vi "Tracer Gas Lite.vi"() -> ()   [LabVIEW 2016]
uses:
  <vilib>/Instr/_visa.llb/VISA Flush IO Buffer Mask.ctl
  <vilib>/Analysis/baseanly.llb/Mean (DBL).vi
  <vilib>/Analysis/NI_AALBase.lvlib
panel:
  in  "Reset AVG":bool
  out "Airflow":waveform(dbl)(graph)
  out "Airflow (SCFM)":dbl
  out "Base GA data":T1
  in  "Tab Control":T2(tab)
  out "CO2 Baseline (PPM)":dbl
  out "B-COMMS?":bool
  in  "Baseline Gas Analyzer COM PORT":refnum<visa-resource-name>
  out "set point (slpm)":dbl
  out "mass flow (slpm)":dbl
  out "CO2 (PPM)":dbl
  out "Inj-comms?":bool
  out "P-COMMS?":bool
  in  "Start new filename":bool
  out "Current time":timestamp format="%<%H:%M:%S>T"
  in  "Shut off injection":bool
  in  "Set point (slpm)":dbl
  in  "Pulse Gas Analyzer COM PORT":refnum<visa-resource-name>
  out "Gas analyzer chart":waveform(dbl)[](graph)
  in  "Reset valves":bool
  in  "Valve 3":bool
  in  "Valve 2":bool
  in  "Valve 1":bool
  in  "Zero now":bool
  in  "Bypass warmup":bool
  out "Zeroing":bool
  out "Warming up":bool
  out "Zero timer":dbl format="%<%H:%M:%S>t"
  out "Warm up timer":dbl format="%<%H:%M:%S>t"
  in  "Injector COM PORT":refnum<visa-resource-name>
  out "path":path
  out "file name":string
  in  "Get Ing AVG":bool
  out "Ing AVG Size":i32
  in  "Get CO2 AVG":bool
  out "CO2 AVG Size":i32
  out "Active Valve":string
  out "Injector chart":waveform(dbl)[](graph)
  in  "Estimated Usable Weight (lbs)":dbl
  out "Estimated test time avialable (hh:mm:ss)":dbl=nan format="%<%H:%M:%S>t"
  in  "Injection rate (slpm)":dbl
  in  "Actual Baseline CO2 Concentration (ppm)":dbl
  in  "Actual Measured CO2 Concentration (ppm)":dbl
  in  "Actual Injection Rate (slpm)":dbl
  out "Calculated Flow (scfm)":dbl
  out "Uncertainty (+/- scfm)":dbl=nan
  out "Uncertainty (%)":dbl=nan
  in  "Ambient CO2 (ppm)":dbl=450.0
  in  "Target CO2 Concentration (ppm)":dbl=1500.0
  in  "Estimated Flow (scfm)":dbl=5000.0
  out "Estimated Injection Rate (slpm)":dbl=148.66204162537164
  in  "Temperature override":bool
  out "Injector status":cluster{"[1]":dbl, "[2]":dbl}(graph)
  out "Gas analyzer status":T3(graph)
  out "Boolean":bool
  out "Inj. options":u16(ring) items=["Default", "Pass Set Point", "Reset"]
  out "Injector warm up":T3(graph)
  out "Gas analyzer warm up":dbl[][](graph)
  in  "Override":bool
  in  "Enum":T4(ring)
  out "Current value":T4(ring)
  out "GA data":T1
  out "injector data":T5
  out "error codes":string
  out "Result path":path
  out "write GA data?":bool
  out "write inj data?":bool
  in  "Temp In Range?":bool
  in  "upper limit":dbl=40.0
  in  "lower limit":dbl=5.0
  # "Calculate injection rate based on baseline CO2, target CO2, and estimated airflow rate."
  # "Time available for testing based on the mass of CO2 inside the tank and the desired injection rate."
  # "Calculate airflow rate and uncertainty based on actual injection rate, baseline CO2, and measured CO2."
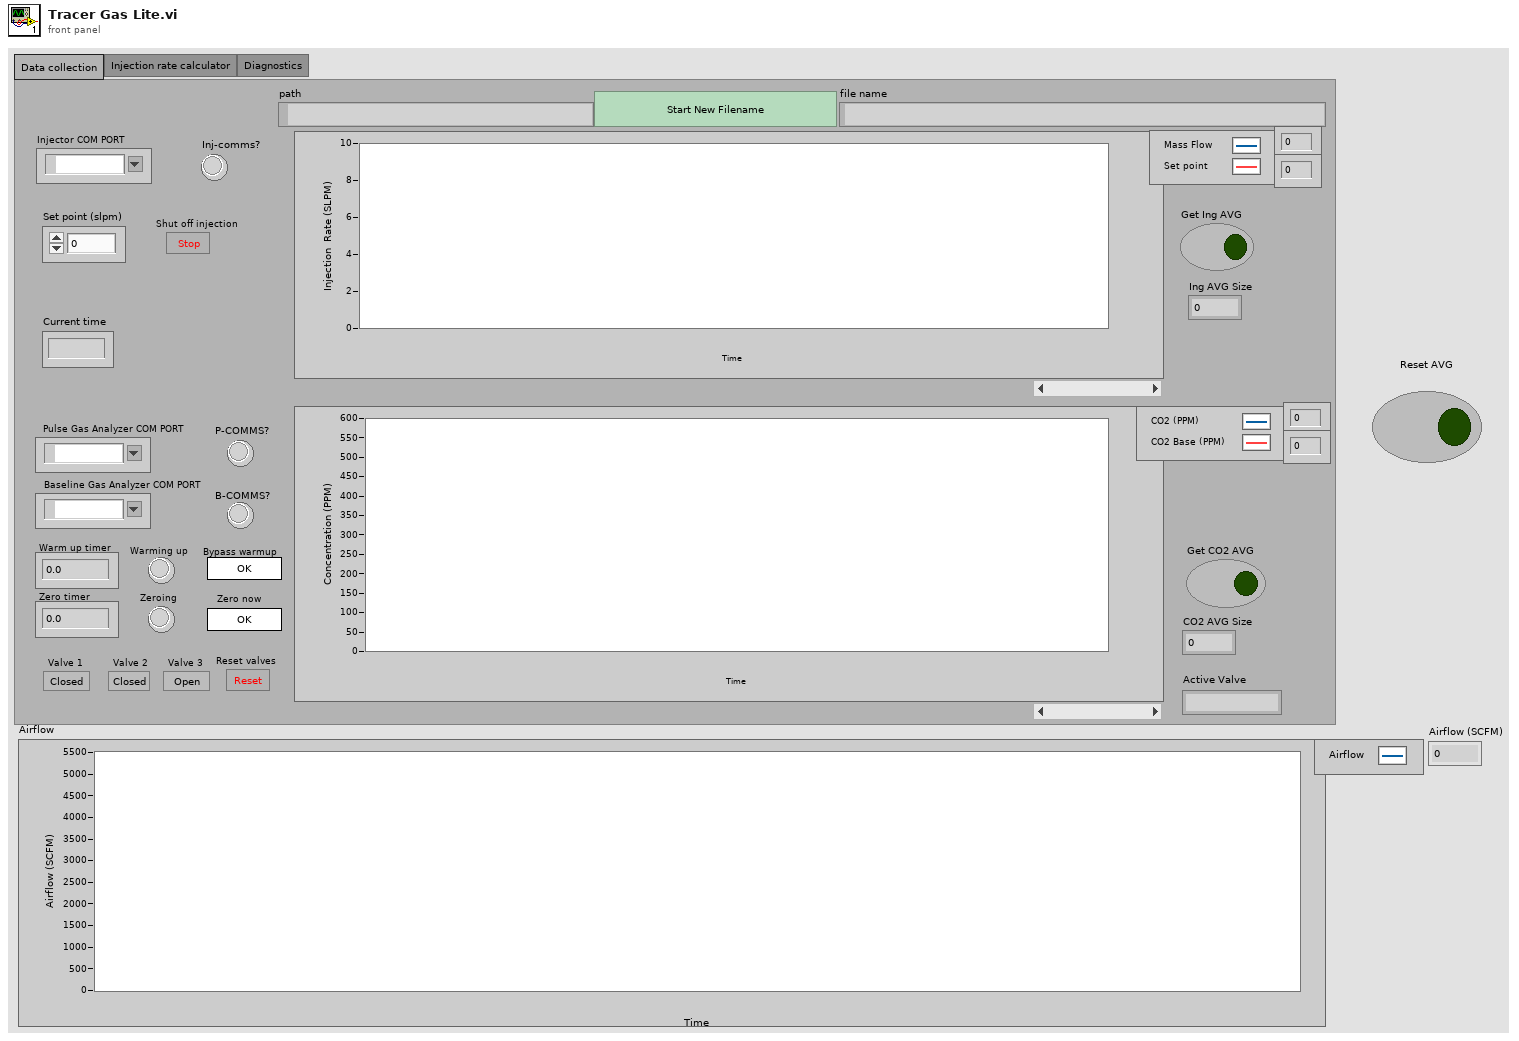
[diagram p1: front panel]
types:
  T1 = cluster{"seconds since 1Jan1904":timestamp, "date string":string, "time string":string, "Array[3]":string, "Array[4]":string, "Array[7]":string, "Array[8]":string, "Array[9]":string}
  T2 = enum32{"Data collection", "Injection rate calculator", "Diagnostics"}
  T3 = cluster{"[0]":dbl, "[1]":dbl, "[2]":dbl, "[3]":dbl, "[4]":dbl, "[5]":dbl, "[6]":dbl, "[7]":dbl, "[8]":dbl}
  T4 = enum16{"Startup", "Warm up", "Poll/Zero", "Run", "Shutdown"}
  T5 = cluster{"seconds since 1Jan1904":timestamp, "date string":string, "time string":string, "[1]":dbl, "[2]":dbl, "[3]":dbl, "[4]":dbl, "[5]":dbl}
  T6 = enum16{"Time", "Zero", "Poll", "Read Buffer", "Set Stream", "Set Poll", "Pump On", "Pump Off", "Set Zero Timing", "Set CO2 Avg.", "Set Measument Format", "Startup Zero Off", "Statup Zero On", "Short Zero Duration", "Set Scaling Factor", "Set Dec Points", "Set Low CO2 Alarm", "Set Analog Output Type", "Set Analog Output Scaling", "Set Data Valid Pin I/O", "Save Current Settings", "Restore Default Settings", "Display Current Settings", "Medium Zero Duration", "Long Zero Duration"}
  T7 = enum16{"Poll", "Set Stream", "Set Poll", "Define Set Point", "Gas Select", "Set P Gain", "Set D Gain", "Get P Gain", "Get D Gain", "Assign New Addess", ""}
  T8 = typedef "VISA Flush IO Buffer Mask.ctl" = u16
  T9 = cluster{"[0]":string, "[1]":string, "[2]":string, "[3]":string, "[4]":string}
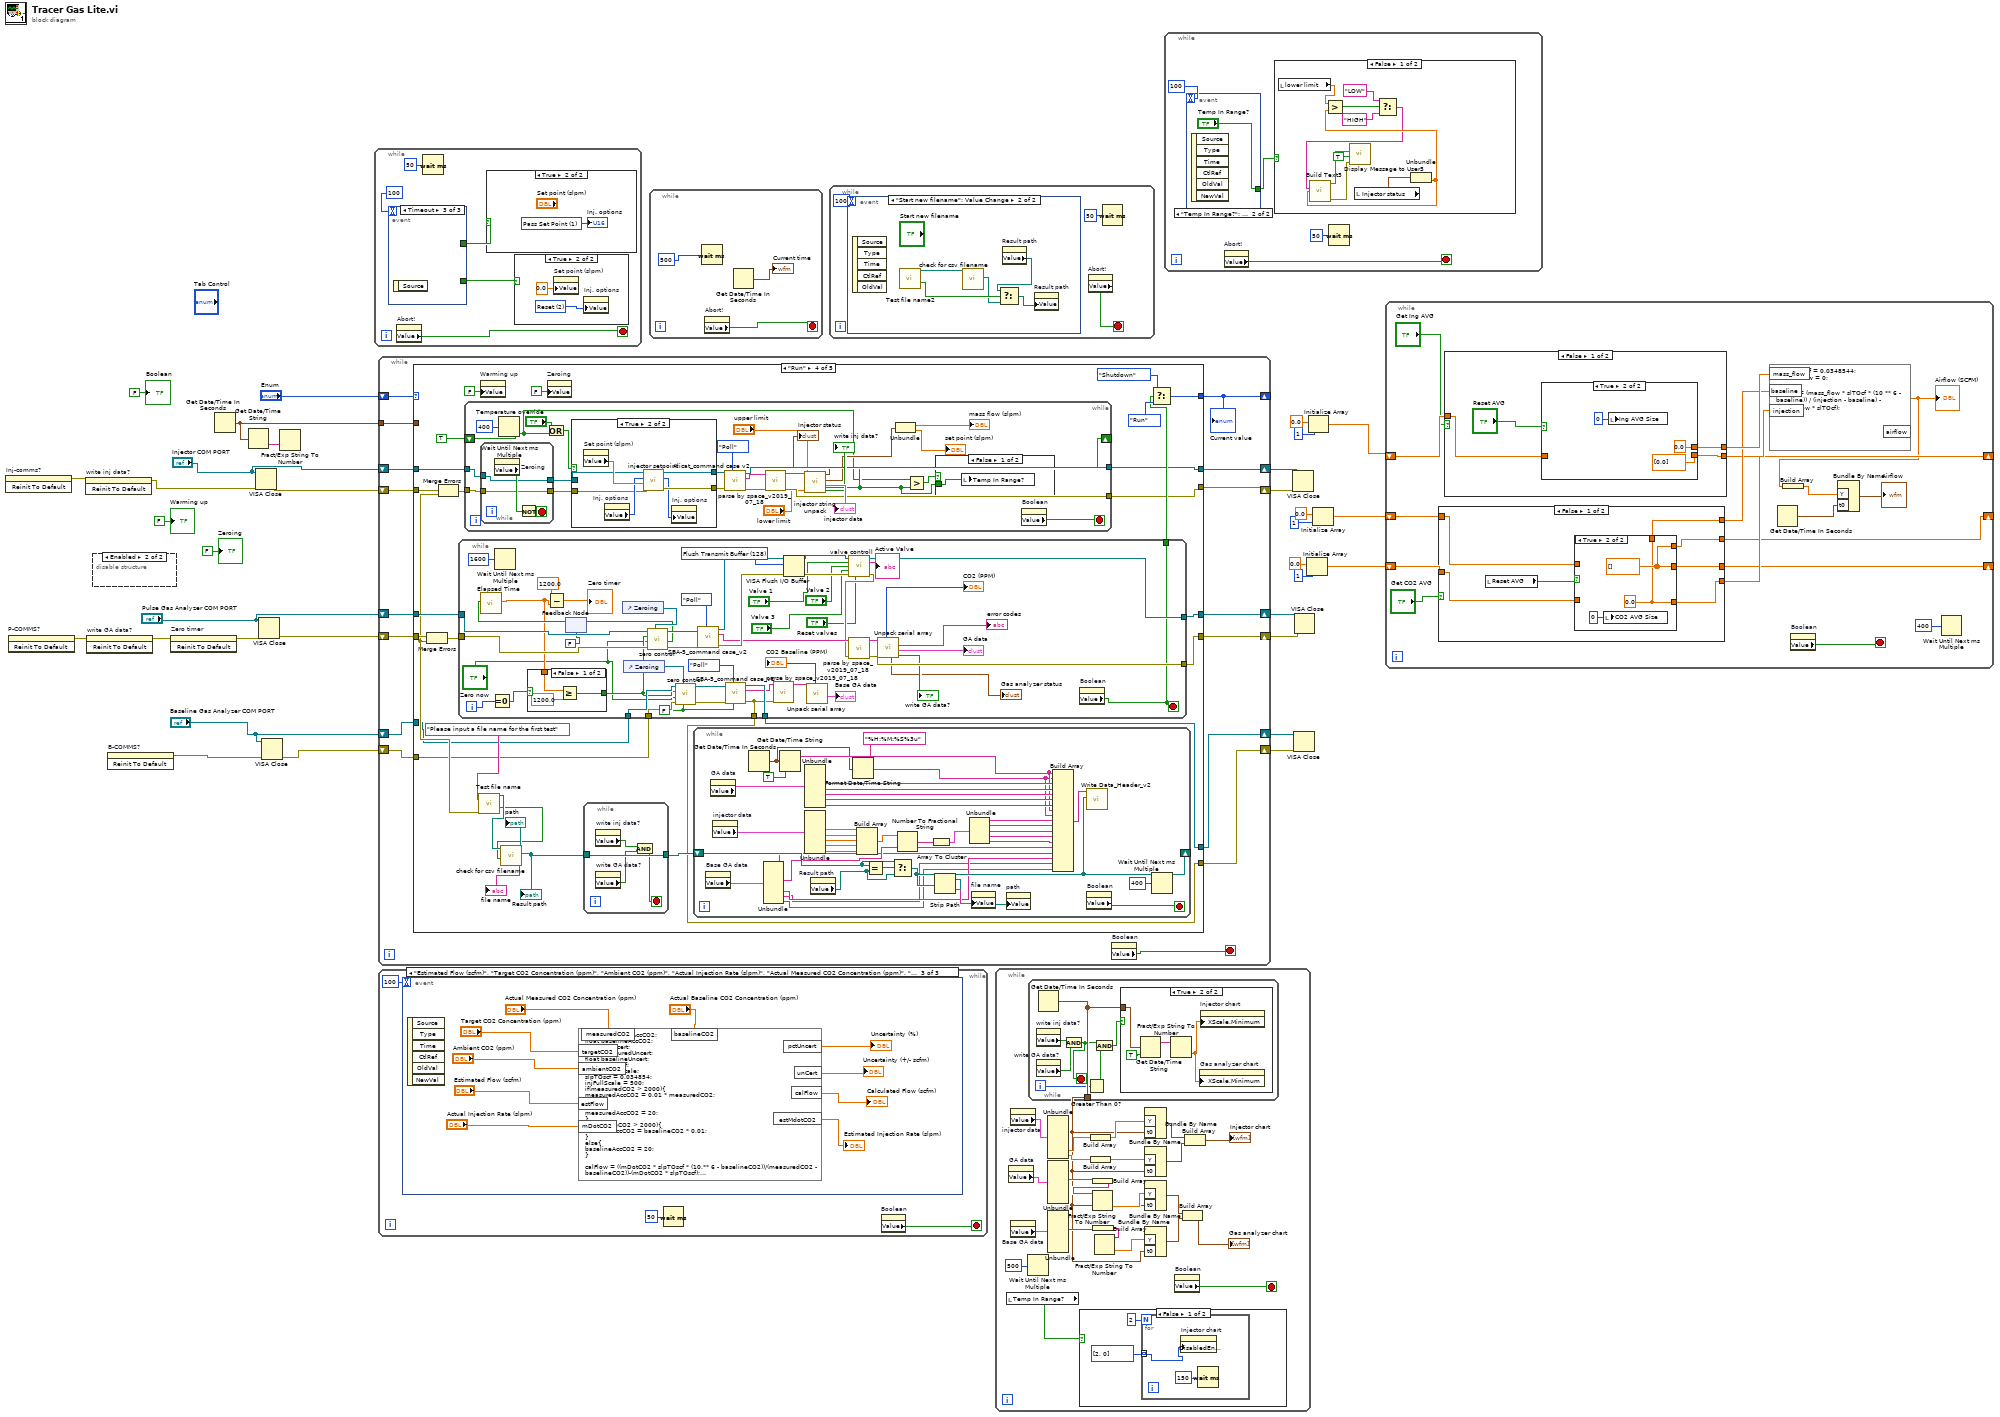
[diagram p0: block diagram]
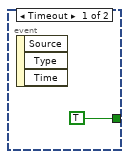
[diagram p3: hidden frame]
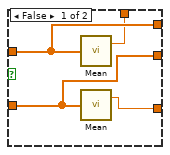
[diagram p4: hidden frame]
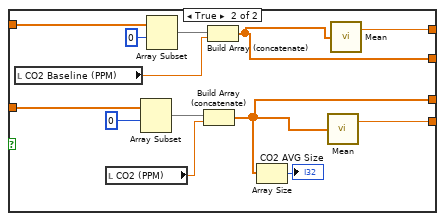
[diagram p5: hidden frame]
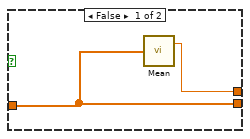
[diagram p6: hidden frame]
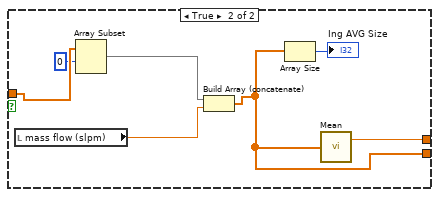
[diagram p7: hidden frame]
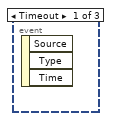
[diagram p10: hidden frame]
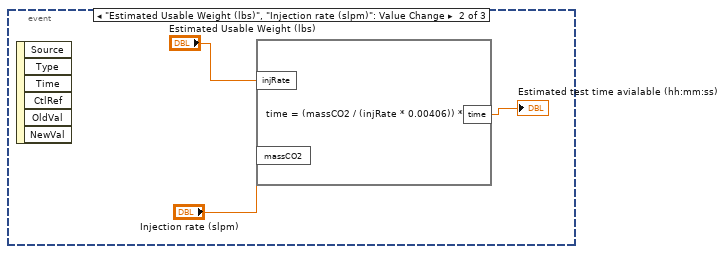
[diagram p11: hidden frame]
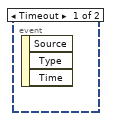
[diagram p12: hidden frame]
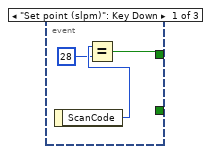
[diagram p15: hidden frame]
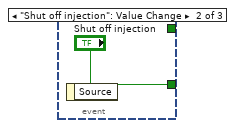
[diagram p16: hidden frame]
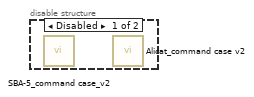
[diagram p17: hidden frame]
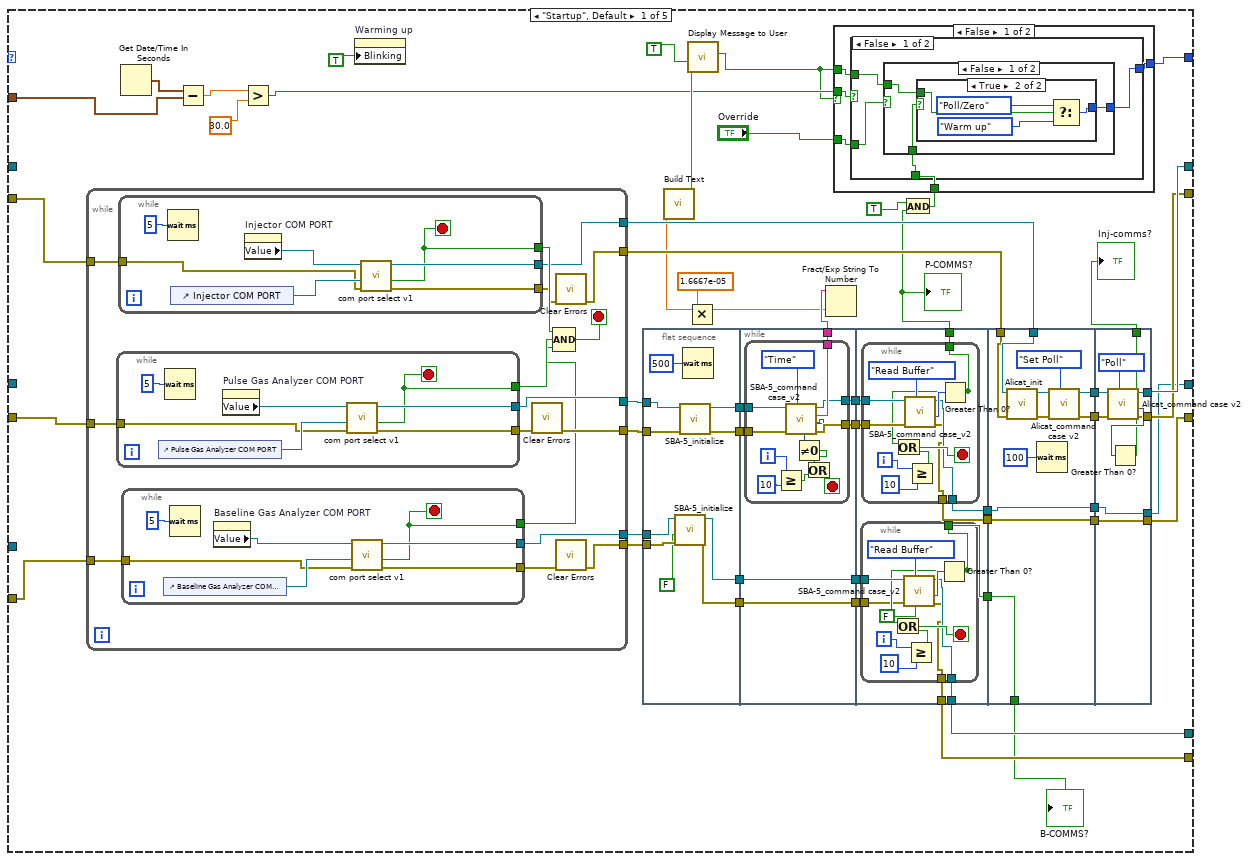
[diagram p18: hidden frame]
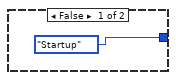
[diagram p19: hidden frame]
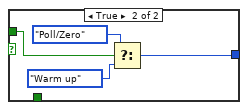
[diagram p20: hidden frame]
diagram:
  n1 = invoke on="Inj-comms?" class="Bool (strict)" method="Reinit To Default"() -> (error out=w16:errorcluster)  [unwired: 3 in, 2 out]
  n2 = invoke on="P-COMMS?" class="Bool (strict)" method="Reinit To Default"() -> (error out=w19:errorcluster)  [unwired: 3 in, 2 out]
  n3 = invoke on="write inj data?" class="Bool (strict)" method="Reinit To Default"(error in=w16) -> (error out=w15:errorcluster)  [unwired: 2 in, 2 out]
  n4 = invoke on="write GA data?" class="Bool (strict)" method="Reinit To Default"(error in=w19) -> (error out=w18:errorcluster)  [unwired: 2 in, 2 out]
  n5 = disable-structure shown="Enabled" {
    frame Disabled {
      n6 = call "SBA-5_command case_v2.vi"() -> ()  [unwired: 8 in, 4 out]
      n7 = call "Alicat_command case v2.vi"() -> ()  [unwired: 8 in, 4 out]
    }
    frame Enabled {
    }
  }
  n8 = invoke on="B-COMMS?" class="Bool (strict)" method="Reinit To Default"() -> (error out=w11:errorcluster)  [unwired: 3 in, 2 out]
  n9 = invoke on="Zero timer" class="DigNum (strict)" method="Reinit To Default"(error in=w18) -> (error out=w17:errorcluster)  [unwired: 2 in, 2 out]
  n10 = Get Date/Time In Seconds() -> (seconds since 1Jan1904=w28:timestamp)
  n11 = Get Date/Time String(seconds (now)=w28) -> (time string=w27:string)  [unwired: 2 in, 1 out]
  n12 = VISA Close(VISA resource name="Injector COM PORT", error in (no error)=w15) -> (error out=w29:errorcluster)
  n13 = VISA Close(VISA resource name="Pulse Gas Analyzer COM PORT", error in (no error)=w17) -> (error out=w32:errorcluster)
  n14 = VISA Close(VISA resource name="Baseline Gas Analyzer COM PORT", error in (no error)=w11) -> (error out=w14:errorcluster)
  n15 = Fract/Exp String To Number(string=w27) -> ()  [unwired: 3 in, 2 out]
  n16 = while {
    stop <- w35 stop-if-true
    n17 = event shown="[2] Timeout" {
      selector: _ -> [_ _ _]
      dyn-events: _ -> [_ _ _]
      timeout: 100 -> [_ _ _]
      tunnel: [_ "Shut off injection" _] -> w37
      tunnel: [w42 _ _] -> w34
      event "Set point (slpm)": Key Down {
        n18 = event-data() -> ("ScanCode"=w44:i16)  [unwired: 1 in]
        n19 = Equal?(x=w44, y=i16 28) -> (x = y?=w42:bool)
      }
      event "Shut off injection": Value Change {
        n20 = event-data() -> ()  [unwired: 1 in, 1 out]
      }
      event Timeout {
        n21 = event-data() -> ()  [unwired: 1 in, 1 out]
      }
    }
    n22 = property on="Abort!" class="Bool (strict)"() -> ("Value"=w35:bool)  [unwired: 2 in, 2 out]
    n23 = Wait (ms)(milliseconds to wait=u32 50) -> ()  [unwired: 1 out]
    n24 = case shown="True" w34 {
      frame False {
      }
      frame True {
        w41 = u16 1 items=["Default", "Pass Set Point", "Reset"] ("Menu Ring")
        "Inj. options" <- w41
      }
    }
    n25 = case shown="True" w37 {
      frame False {
      }
      frame True {
        w40 = u16 2 items=["Default", "Pass Set Point", "Reset"] ("Menu Ring")
        n26 = property on="Set point (slpm)" class="DigNum (strict)"("Value"=0.0 ("Set point (slpm)")) -> ()  [unwired: 2 in, 2 out]
        n27 = property on="Inj. options" class="Ring (strict)"("Value"=w40) -> ()  [unwired: 2 in, 2 out]
      }
    }
  }
  n28 = while {
    shift-right: [w57] -> w24
    shift-left: "Pulse Gas Analyzer COM PORT" -> [w60]
    shift-right: [w56] -> w23
    shift-left: w32 -> [w59]
    shift-right: [w58] -> w26
    shift-left: "Injector COM PORT" -> [w55]
    shift-right: [w51] -> _
    shift-left: "Enum" -> [w61]
    shift-right: [w53] -> w25
    shift-left: w29 -> [w54]
    tunnel: w28 -> [w52]
    shift-right: [w47] -> w13
    shift-left: "Baseline Gas Analyzer COM PORT" -> [w49]
    shift-right: [w46] -> w12
    shift-left: w14 -> [w48]
    stop <- w50 stop-if-true
    n29 = case shown="\"Run\"" w61 {
      tunnel: w60 -> [_ w283 w337 w406 w558]
      tunnel: w59 -> [w111 w286 w340 w394 w557]
      tunnel: [w95 w276 w346 w384 w556] -> w58
      tunnel: [w94 w277 w345 w385 w555] -> w53
      tunnel: [w69 w274 w338 w404 w558] -> w57
      tunnel: [w66 w275 w334 w405 w557] -> w56
      tunnel: w55 -> [_ w281 w346 w397 w556]
      tunnel: w54 -> [w101 w282 w345 w396 w555]
      tunnel: w52 -> [w92 _ _ _ _]
      tunnel: [w88 T4."Poll/Zero" ("Enum") T4."Run" ("Enum") w400 T4."Shutdown" ("Enum")] -> w51
      tunnel: w49 -> [_ w272 w332 w382 w554]
      tunnel: w48 -> [w78 w271 w331 w381 w553]
      tunnel: [w65 w269 w330 w380 w554] -> w47
      tunnel: [w64 w270 w329 w379 w553] -> w46
      frame "Startup", Default {
        n30 = while {
          tunnel: [w240] -> w104
          tunnel: w111 -> [w245]
          tunnel: [w241] -> w105
          tunnel: [w239] -> w110
          tunnel: [w238] -> w109
          tunnel: w101 -> [w237]
          tunnel: w78 -> [w236]
          tunnel: [w233] -> w77
          tunnel: [w232] -> w76
          stop <- w247 stop-if-true
          n31 = while {
            tunnel: [w268] -> w246
            tunnel: w245 -> [w264]
            tunnel: [w263] -> w238
            tunnel: [w262] -> w242
            stop <- w262 stop-if-true
            n32 = control-ref of="Pulse Gas Analyzer COM PORT"() -> (w266:refnum<vi>)
            n33 = Wait (ms)(milliseconds to wait=u32 5) -> ()  [unwired: 1 out]
            n34 = property on="Pulse Gas Analyzer COM PORT" class="VISAName"() -> ("Value"=w265:refnum<visa-resource-name>)  [unwired: 2 in, 2 out]
            n35 = call "com port select v1.vi"("error in (no error)"=w264, "Ctl Refnum"=w266, "VISA resource name in"=w265) -> ("error out"=w268:errorcluster, "COM PORT?"=w262:bool, "VISA resource name out"=w263:refnum<visa-resource-name>)  [unwired: 6 in]
          }
          n36 = while {
            tunnel: [w258] -> w243
            tunnel: [w257] -> w241
            tunnel: [w256] -> w244
            tunnel: w237 -> [w255]
            stop <- w256 stop-if-true
            n37 = Wait (ms)(milliseconds to wait=u32 5) -> ()  [unwired: 1 out]
            n38 = control-ref of="Injector COM PORT"() -> (w261:refnum<vi>)
            n39 = property on="Injector COM PORT" class="VISAName"() -> ("Value"=w259:refnum<visa-resource-name>)  [unwired: 2 in, 2 out]
            n40 = call "com port select v1.vi"("error in (no error)"=w255, "Ctl Refnum"=w261, "VISA resource name in"=w259) -> ("error out"=w258:errorcluster, "COM PORT?"=w256:bool, "VISA resource name out"=w257:refnum<visa-resource-name>)  [unwired: 6 in]
          }
          n41 = while {
            tunnel: [w254] -> w235
            tunnel: w236 -> [w251]
            tunnel: [w250] -> w233
            tunnel: [w249] -> w234
            stop <- w249 stop-if-true
            n42 = control-ref of="Baseline Gas Analyzer COM PORT"() -> (w252:refnum<vi>)
            n43 = Wait (ms)(milliseconds to wait=u32 5) -> ()  [unwired: 1 out]
            n44 = property on="Baseline Gas Analyzer COM PORT" class="VISAName"() -> ("Value"=w248:refnum<visa-resource-name>)  [unwired: 2 in, 2 out]
            n45 = call "com port select v1.vi"("error in (no error)"=w251, "Ctl Refnum"=w252, "VISA resource name in"=w248) -> ("error out"=w254:errorcluster, "COM PORT?"=w249:bool, "VISA resource name out"=w250:refnum<visa-resource-name>)  [unwired: 6 in]
          }
          n46 = call <vilib>:"Clear Errors.vi"("error in (no error)"=w246) -> ("error out"=w239:errorcluster)  [unwired: 5 in, 1 out]
          n47 = Compound Arithmetic op=AND(w244, w242, w234) -> (w247:bool)
          n48 = call <vilib>:"Clear Errors.vi"("error in (no error)"=w243) -> ("error out"=w240:errorcluster)  [unwired: 5 in, 1 out]
          n49 = call <vilib>:"Clear Errors.vi"("error in (no error)"=w235) -> ("error out"=w232:errorcluster)  [unwired: 5 in, 1 out]
        }
        n50 = Get Date/Time In Seconds() -> (seconds since 1Jan1904=w93:timestamp)
        n51 = Subtract(x=w93, y=w92) -> (x-y=w91:dbl)
        n52 = Greater?(x=w91, y=30.0) -> (0:w89:bool)
        n53 = property on="Warming up" class="Bool (strict)"("Blinking"=TRUE) -> ()  [unwired: 2 in, 2 out]
        n54 = flat-sequence {
          tunnel: w110 -> [w159]
          tunnel: w109 -> [w158]
          tunnel: [w156] -> w108
          tunnel: [w155] -> w107
          tunnel: w77 -> [w154]
          tunnel: w76 -> [w153]
          tunnel: [w152] -> w74
          tunnel: [w151] -> w72
          tunnel: w108 -> [w166]
          tunnel: w107 -> [w165]
          tunnel: [w164] -> w103
          tunnel: [w163] -> w100
          tunnel: [w162] -> w99
          tunnel: [w161] -> w75
          tunnel: w74 -> [w161]
          tunnel: [w160] -> w73
          tunnel: w72 -> [w160]
          tunnel: w100 -> [w188]
          tunnel: w99 -> [w187]
          tunnel: [w186] -> w79
          tunnel: w75 -> [w185]
          tunnel: w73 -> [w184]
          tunnel: [w183] -> w70
          tunnel: [w182] -> w67
          tunnel: [w181] -> w65
          tunnel: [w180] -> w64
          tunnel: [w179] -> w62
          tunnel: w105 -> [w222]
          tunnel: w104 -> [w221]
          tunnel: [w219] -> w97
          tunnel: [w220] -> w96
          tunnel: [w214] -> w71
          tunnel: w70 -> [w214]
          tunnel: [w213] -> w68
          tunnel: w67 -> [w213]
          tunnel: [w212] -> w63
          tunnel: w62 -> [w212]
          tunnel: w97 -> [w230]
          tunnel: w96 -> [w231]
          tunnel: [w227] -> w80
          tunnel: [w226] -> w95
          tunnel: [w225] -> w94
          tunnel: w71 -> [w224]
          tunnel: [w224] -> w69
          tunnel: w68 -> [w223]
          tunnel: [w223] -> w66
          frame #0 {
            n55 = call "SBA-5_initialize.vi"("error in (no error)"=w153, "Valve control"=FALSE, "VISA resource name"=w154) -> ("error out"=w151:errorcluster, "VISA resource name out"=w152:refnum<visa-resource-name>)  [unwired: 7 in]
            n56 = call "SBA-5_initialize.vi"("error in (no error)"=w159, "VISA resource name"=w158) -> ("error out"=w155:errorcluster, "VISA resource name out"=w156:refnum<visa-resource-name>)  [unwired: 8 in]
            n57 = Wait (ms)(milliseconds to wait=u32 500) -> ()  [unwired: 1 out]
          }
          frame #1 {
            n58 = while {
              tunnel: w166 -> [w177]
              tunnel: w165 -> [w176]
              tunnel: [w175] -> w164
              tunnel: [w174] -> w163
              tunnel: [w173] -> w162
              i -> [w172]
              stop <- w167 stop-if-true
              n59 = Greater Or Equal?(x=w172, y=10) -> (x >= y?=w170:bool)
              n60 = call "SBA-5_command case_v2.vi"("Case"=T6."Time", "error in (no error)"=w176, "VISA resource name"=w177) -> ("error out"=w173:errorcluster, "bytes out"=w168:u32, "StringFromSBA-5"=w175:string, "dup VISA resource name"=w174:refnum<visa-resource-name>)  [unwired: 5 in]
              n61 = Not Equal To 0?(x=w168) -> (x != 0?=w169:bool)
              n62 = Or(x=w169, y=w170) -> (x .or. y?=w167:bool)
            }
          }
          frame #2 {
            n63 = while {
              tunnel: w185 -> [w199]
              tunnel: [w193] -> w179
              tunnel: [w192] -> w181
              tunnel: [w191] -> w180
              tunnel: w184 -> [w190]
              i -> [w196]
              stop <- w197 stop-if-true
              n64 = call "SBA-5_command case_v2.vi"("Valve control"=FALSE, "Case"=T6."Read Buffer", "error in (no error)"=w190, "VISA resource name"=w199) -> ("error out"=w191:errorcluster, "bytes out"=w198:u32, "dup VISA resource name"=w192:refnum<visa-resource-name>)  [unwired: 4 in, 1 out]
              n65 = Greater Or Equal?(x=w196, y=10) -> (x >= y?=w194:bool)
              n66 = Greater Than 0?(x=w198) -> (x > 0?=w193:bool)
              n67 = Or(x=w193, y=w194) -> (x .or. y?=w197:bool)
            }
            n68 = while {
              tunnel: w188 -> [w210]
              tunnel: w187 -> [w209]
              tunnel: [w203] -> w186
              tunnel: [w202] -> w183
              tunnel: [w201] -> w182
              i -> [w206]
              stop <- w207 stop-if-true
              n69 = call "SBA-5_command case_v2.vi"("Case"=T6."Read Buffer", "error in (no error)"=w209, "VISA resource name"=w210) -> ("error out"=w201:errorcluster, "bytes out"=w208:u32, "dup VISA resource name"=w202:refnum<visa-resource-name>)  [unwired: 5 in, 1 out]
              n70 = Greater Or Equal?(x=w206, y=10) -> (x >= y?=w204:bool)
              n71 = Greater Than 0?(x=w208) -> (x > 0?=w203:bool)
              n72 = Or(x=w203, y=w204) -> (x .or. y?=w207:bool)
            }
          }
          frame #3 {
            n73 = call "Alicat_init.vi"("error in (no error)"=w221, "VISA resource name"=w222) -> ("error out"=w217:errorcluster, "VISA resource name out"=w218:refnum<visa-resource-name>)  [unwired: 8 in]
            n74 = Wait (ms)(milliseconds to wait=u32 100) -> ()  [unwired: 1 out]
            n75 = call "Alicat_command case v2.vi"("Case"=T7."Set Poll", "error in (no error)"=w217, "VISA resource name"=w218) -> ("error out"=w220:errorcluster, "dup VISA resource name"=w219:refnum<visa-resource-name>)  [unwired: 5 in, 2 out]
          }
          frame #4 {
            n76 = call "Alicat_command case v2.vi"("Case"=T7."Poll", "error in (no error)"=w231, "VISA resource name"=w230) -> ("error out"=w225:errorcluster, "bytes at port"=w228:u32, "dup VISA resource name"=w226:refnum<visa-resource-name>)  [unwired: 5 in, 1 out]
            n77 = Greater Than 0?(x=w228) -> (x > 0?=w227:bool)
          }
        }
        n78 = Fract/Exp String To Number(string=w103) -> (number=w102:dbl)  [unwired: 3 in, 1 out]
        n79 = Multiply(x=w102, y=1.6667e-05) -> (x*y=w84:dbl)
        n80 = call "Build Text"("minutes"=w84) -> ("Result"=w98:string)  [unwired: 13 in, 1 out]
        n81 = call "Display Message to User"("Enable"=TRUE, "Message"=w98) -> ("Yes"=w81:bool)  [unwired: 8 in, 1 out]
        n82 = And(x=TRUE, y=w79) -> (x .and. y?=w86:bool)
        n83 = case shown="False" w81 {
          tunnel: w89 -> [w116 _]
          tunnel: [w115 T4."Poll/Zero" ("Enum")] -> w88
          tunnel: "Override" -> [w114 _]
          tunnel: w81 -> [w113 _]
          tunnel: w86 -> [w112 _]
          frame False {
            n84 = case shown="False" w116 {
              tunnel: [w118 w134] -> w115
              tunnel: w114 -> [w120 w136]
              tunnel: w113 -> [w119 w135]
              tunnel: w112 -> [w117 w133]
              frame False {
                n85 = case shown="False" w120 {
                  tunnel: w119 -> [w122 w131]
                  tunnel: [w121 w129] -> w118
                  tunnel: w117 -> [w123 _]
                  frame False {
                    n86 = case shown="True" w123 {
                      tunnel: w122 -> [_ w128]
                      tunnel: [T4."Startup" ("Enum") w125] -> w121
                      frame False {
                      }
                      frame True {
                        n87 = Select(t=T4."Poll/Zero" ("Enum"), s=w128, f=T4."Warm up" ("Enum")) -> (s? t:f=w125:T4)
                      }
                    }
                  }
                  frame True {
                    n88 = Select(t=T4."Poll/Zero" ("Enum"), s=w131, f=T4."Warm up" ("Enum")) -> (s? t:f=w129:T4)
                  }
                }
              }
              frame True {
                n89 = case shown="True" w136 {
                  tunnel: w135 -> [w138 w148]
                  tunnel: [w137 w145] -> w134
                  tunnel: w133 -> [w139 _]
                  frame False {
                    n90 = case shown="False" w139 {
                      tunnel: w138 -> [_ w142]
                      tunnel: [T4."Shutdown" ("Enum") w141] -> w137
                      frame False {
                      }
                      frame True {
                        n91 = Select(t=T4."Poll/Zero" ("Enum"), s=w142, f=T4."Warm up" ("Enum")) -> (s? t:f=w141:T4)
                      }
                    }
                  }
                  frame True {
                    n92 = Select(t=T4."Poll/Zero" ("Enum"), s=w148, f=T4."Warm up" ("Enum")) -> (s? t:f=w145:T4)
                  }
                }
              }
            }
          }
          frame True {
          }
        }
        "Inj-comms?" <- w80
        "P-COMMS?" <- w79
        "B-COMMS?" <- w63
      }
      frame "Warm up" {
        n93 = property on="Warm up timer" class="DigNum (strict)"(error in=w286, "Value"=900.0 ("Warm up timer")) -> (error out=w284:errorcluster)  [unwired: 1 in, 1 out]
        n94 = property on="Warming up" class="Bool (strict)"("Blinking"=FALSE) -> (error out=w279:errorcluster)  [unwired: 2 in, 1 out]
        n95 = while {
          tunnel: w284 -> [w317]
          tunnel: w283 -> [w318]
          tunnel: w282 -> [w315]
          tunnel: w281 -> [w314]
          tunnel: [w303] -> w276
          tunnel: [w301] -> w277
          tunnel: [w300] -> w275
          tunnel: [w299] -> w274
          tunnel: w272 -> [w298]
          tunnel: w271 -> [w297]
          tunnel: [w290] -> w269
          tunnel: [w289] -> w270
          stop <- w311 stop-if-true
          n96 = Wait Until Next ms Multiple(millisecond multiple=u32 1600) -> ()  [unwired: 1 out]
          n97 = call "SBA-5_command case_v2.vi"("Case"=T6."Read Buffer", "error in (no error)"=w317, "VISA resource name"=w318) -> ("error out"=w309:errorcluster, "StringFromSBA-5"=w310:string, "dup VISA resource name"=w299:refnum<visa-resource-name>)  [unwired: 5 in, 1 out]
          n98 = call "SBA-5_command case_v2.vi"("Valve control"=FALSE, "Case"=T6."Read Buffer", "error in (no error)"=w297, "VISA resource name"=w298) -> ("error out"=w296:errorcluster, "StringFromSBA-5"=w295:string, "dup VISA resource name"=w290:refnum<visa-resource-name>)  [unwired: 4 in, 1 out]
          n99 = call "Alicat_command case v2.vi"("Case"=T7."Poll", "error in (no error)"=w315, "VISA resource name"=w314) -> ("error out"=w302:errorcluster, "String From Alicat"=w305:string, "dup VISA resource name"=w303:refnum<visa-resource-name>)  [unwired: 5 in, 1 out]
          n100 = call "parse by space_v2019_07_18.vi"("error in (no error)"=w296, "String"=w295) -> ("error out"=w289:errorcluster, "Array"=w294:string[])  [unwired: 8 in]
          n101 = call "parse by space_v2019_07_18.vi"("error in (no error)"=w302, "String"=w305) -> ("error out"=w301:errorcluster, "Array"=w306:string[])  [unwired: 8 in]
          n102 = call "parse by space_v2019_07_18.vi"("error in (no error)"=w309, "String"=w310) -> ("error out"=w300:errorcluster, "Array"=w308:string[])  [unwired: 8 in]
          n103 = Fract/Exp String To Number(string=w306) -> (number=w307:dbl[])  [unwired: 3 in, 1 out]
          n104 = Fract/Exp String To Number(string=w294) -> (number=w292:dbl[])  [unwired: 3 in, 1 out]
          n105 = Fract/Exp String To Number(string=w308) -> (number=w293:dbl[])  [unwired: 3 in, 1 out]
          n106 = Array To Cluster(array=w307) -> (cluster=→"Injector warm up":T3)
          n107 = Build Array(w293, w292) -> (→"Gas analyzer warm up":dbl[][])
          n108 = property on="Warm up timer" class="DigNum (strict)"() -> ("Value"=w312:dbl)  [unwired: 2 in, 2 out]
          n109 = Less Or Equal To 0?(x=w312) -> (x <= 0?=w311:bool)
        }
        n110 = property on="Warming up" class="Bool (strict)"(error in=w279, "Value"=TRUE ("Blinking")) -> ()  [unwired: 1 in, 2 out]
        n111 = while {
          stop <- w323 stop-if-true
          n112 = call "Warm up timing"() -> ("Elapsed Time (s)"=w327:dbl, "Time has Elapsed"=w322:bool)  [unwired: 12 in, 6 out]
          n113 = Wait Until Next ms Multiple(millisecond multiple=u32 500) -> ()  [unwired: 1 out]
          n114 = Compound Arithmetic op=OR(w322, "Bypass warmup") -> (w323:bool)
          n115 = Subtract(x=900.0, y=w327) -> (x-y=w325:dbl)
          n116 = Select(t=0.0, s="Bypass warmup", f=w325) -> (s? t:f=→"Warm up timer":dbl)
        }
      }
      frame "Poll/Zero" {
        n117 = property on="Zeroing" class="Bool (strict)"(error in=w340, "Blinking"=TRUE ("Zeroing")) -> (error out=w336:errorcluster)  [unwired: 1 in, 1 out]
        n118 = property on="Warming up" class="Bool (strict)"("Blinking"=FALSE) -> (error out=w342:errorcluster)  [unwired: 2 in, 1 out]
        n119 = property on="Warming up" class="Bool (strict)"(error in=w342, "Value"=FALSE ("Blinking")) -> ()  [unwired: 1 in, 2 out]
        n120 = while {
          tunnel: w337 -> [w367]
          tunnel: w336 -> [w365]
          tunnel: [w375] -> w338
          tunnel: [w374] -> w335
          i -> [w370]
          stop <- w371 stop-if-true
          n121 = call "SBA-5_command case_v2.vi"("Case"=T6."Set Poll", "error in (no error)"=w365, "VISA resource name"=w367) -> ("error out"=w364:errorcluster, "dup VISA resource name"=w366:refnum<visa-resource-name>)  [unwired: 5 in, 2 out]
          n122 = Wait Until Next ms Multiple(millisecond multiple=u32 1600) -> ()  [unwired: 1 out]
          n123 = call "SBA-5_command case_v2.vi"("Case"=T6."Poll", "error in (no error)"=w364, "VISA resource name"=w366) -> ("error out"=w374:errorcluster, "bytes out"=w376:u32, "dup VISA resource name"=w375:refnum<visa-resource-name>)  [unwired: 5 in, 1 out]
          n124 = Greater?(x=w370, y=5) -> (0:w368:bool)
          n125 = Greater Than 0?(x=w376) -> (x > 0?=w363:bool)
          n126 = property on="P-COMMS?" class="Bool (strict)"("Value"=w363) -> ()  [unwired: 2 in, 2 out]
          n127 = Or(x=w363, y=w368) -> (x .or. y?=w371:bool)
        }
        n128 = while {
          tunnel: w332 -> [w352]
          tunnel: w331 -> [w350]
          tunnel: [w360] -> w330
          tunnel: [w359] -> w329
          i -> [w355]
          stop <- w356 stop-if-true
          w347 = FALSE ("Valve control")
          n129 = call "SBA-5_command case_v2.vi"("Valve control"=w347, "Case"=T6."Set Poll", "error in (no error)"=w350, "VISA resource name"=w352) -> ("error out"=w349:errorcluster, "dup VISA resource name"=w351:refnum<visa-resource-name>)  [unwired: 4 in, 2 out]
          n130 = Wait Until Next ms Multiple(millisecond multiple=u32 1600) -> ()  [unwired: 1 out]
          n131 = call "SBA-5_command case_v2.vi"("Valve control"=w347, "Case"=T6."Poll", "error in (no error)"=w349, "VISA resource name"=w351) -> ("error out"=w359:errorcluster, "bytes out"=w361:u32, "dup VISA resource name"=w360:refnum<visa-resource-name>)  [unwired: 4 in, 1 out]
          n132 = Greater?(x=w355, y=5) -> (0:w353:bool)
          n133 = Greater Than 0?(x=w361) -> (x > 0?=w348:bool)
          n134 = property on="B-COMMS?" class="Bool (strict)"("Value"=w348) -> ()  [unwired: 2 in, 2 out]
          n135 = Or(x=w348, y=w353) -> (x .or. y?=w356:bool)
        }
        n136 = property on="Zeroing" class="Bool (strict)"(error in=w335, "Blinking"=FALSE) -> (error out=w334:errorcluster)  [unwired: 1 in, 1 out]
      }
      frame "Run" {
        n137 = call "Test file name"("prompt"="Please input a file name for the first test") -> ("selected path"=w390:path, "cancelled"=w383:bool, "error out"=w392:errorcluster)  [unwired: 11 in, 1 out]
        n138 = Merge Errors(w394, w392) -> (w393:errorcluster)
        n139 = Merge Errors(w396, w392) -> (w395:errorcluster)
        n140 = while {
          tunnel: w406 -> [w546]
          tunnel: w393 -> [w545]
          tunnel: [w535] -> w405
          tunnel: [w524] -> w404
          tunnel: [w516] -> w401
          tunnel: w382 -> [w513]
          tunnel: w381 -> [w512]
          tunnel: [w503] -> w380
          tunnel: [w502] -> w379
          i -> [w529]
          stop <- w516 stop-if-true
          w500 = FALSE ("Valve control")
          w538 = T8 128 items=["Flush Receive Buffer"=16, "Write Transmit Buffer to Device"=32, "Flush Receive Buffer (No I/O)"=64, "Flush Transmit Buffer"=128] ("Mask")
          n141 = Equal To 0?(x=w529) -> (x = 0?=w528:bool)
          n142 = Wait Until Next ms Multiple(millisecond multiple=u32 1600) -> ()  [unwired: 1 out]
          n143 = feedback #1(FALSE ("Zero reset")) -> (w532:bool)
          n144 = call "Elapsed Time"("Reset"=w532) -> ("Elapsed Time (s)"=w530:dbl)  [unwired: 11 in, 7 out]
          n145 = case shown="False" w528 {
            tunnel: w530 -> [w550 _]
            tunnel: [w549 TRUE] -> w511
            frame False {
              n146 = Greater Or Equal?(x=w550, y=1200.0) -> (x >= y?=w549:bool)
            }
            frame True {
            }
          }
          n147 = Subtract(x=1200.0, y=w530) -> (x-y=→"Zero timer":dbl)
          n148 = control-ref of="Zeroing"() -> (w544:refnum<vi>)
          n149 = control-ref of="Zeroing"() -> (w501:refnum<vi>)
          n150 = call "zero control.vi"("Ctl Refnum"=w544, "error in (no error)"=w545, "Zero now"="Zero now", "Zero timer"=w511, "VISA resource name"=w546) -> ("error out"=w542:errorcluster, "Zero reset"=w533:bool, "VISA resource out"=w543:refnum<visa-resource-name>)  [unwired: 4 in]
          n151 = feedback-in #1(w533) -> ()
          n152 = call "zero control.vi"("Valve control"=w500, "Ctl Refnum"=w501, "error in (no error)"=w512, "Zero now"="Zero now", "Zero timer"=w511, "VISA resource name"=w513) -> ("error out"=w508:errorcluster, "VISA resource out"=w509:refnum<visa-resource-name>)  [unwired: 3 in, 1 out]
          n153 = call "SBA-5_command case_v2.vi"("Case"=T6."Poll", "error in (no error)"=w542, "VISA resource name"=w543) -> ("error out"=w539:errorcluster, "StringFromSBA-5"=w537:string, "dup VISA resource name"=w540:refnum<visa-resource-name>)  [unwired: 5 in, 1 out]
          n154 = call "SBA-5_command case_v2.vi"("Valve control"=w500, "Case"=T6."Poll", "error in (no error)"=w508, "VISA resource name"=w509) -> ("error out"=w502:errorcluster, "StringFromSBA-5"=w499:string, "dup VISA resource name"=w503:refnum<visa-resource-name>)  [unwired: 4 in, 1 out]
          n155 = call "parse by space_v2019_07_18.vi"("error in (no error)"=w502, "String"=w499) -> ("Array"=w506:string[])  [unwired: 8 in, 1 out]
          n156 = VISA Flush I/O Buffer(VISA resource name=w540, mask (16)=w538, error in (no error)=w539) -> (VISA resource name out=w527:refnum<visa-resource-name>, error out=w526:errorcluster)
          n157 = call "Unpack serial array.vi"("Array"=w506) -> ("Cluster 2"=→"Base GA data":T1, "Numeric"=→"CO2 Baseline (PPM)":i32)  [unwired: 4 in, 5 out]
          n158 = call "valve controll.vi"("VISA Refnum in"=w527, "Valve 1"="Valve 1", "Valve 2"="Valve 2", "Valve 3"="Valve 3", "error in (no error)"=w526, "Reset valves"="Reset valves") -> ("VISA Refnum in 2"=w524:refnum<visa-resource-name>, "Active Valve"=→"Active Valve":string, "error out"=w525:errorcluster)  [unwired: 7 in]
          n159 = call "parse by space_v2019_07_18.vi"("error in (no error)"=w525, "String"=w537) -> ("error out"=w535:errorcluster, "Array"=w536:string[])  [unwired: 8 in]
          n160 = call "Unpack serial array.vi"("Array"=w536) -> ("write data?"=→"write GA data?":bool, "Cluster 2"=→"GA data":T1, "Array[10]"=→"error codes":string, "Cluster"=→"Gas analyzer status":T3, "Numeric"=→"CO2 (PPM)":i32)  [unwired: 4 in, 2 out]
          n161 = property on="Boolean" class="Bool (strict)"() -> ("Value"=w516:bool)  [unwired: 2 in, 2 out]
        }
        n162 = while {
          tunnel: w397 -> [w468]
          tunnel: w395 -> [w466]
          tunnel: [w464] -> w385
          tunnel: [w463] -> w384
          shift-right: [w452] -> _
          shift-left: TRUE -> [w451]
          stop <- w462 stop-if-true
          n163 = while {
            tunnel: w468 -> [w495]
            tunnel: [w495] -> w467
            tunnel: w466 -> [w494]
            tunnel: [w494] -> w465
            stop <- w496 stop-if-true
            n164 = property on="Zeroing" class="Bool (strict)"() -> ("Value"=w497:bool)  [unwired: 2 in, 2 out]
            n165 = Not(x=w497) -> (.not. x?=w496:bool)
          }
          n166 = Wait Until Next ms Multiple(millisecond multiple=u32 400) -> ()  [unwired: 1 out]
          n167 = Or(x="Temperature override", y=w451) -> (x .or. y?=w454:bool)
          n168 = case shown="True" w454 {
            tunnel: [w485 w492] -> w476
            tunnel: [w484 w491] -> w475
            tunnel: w467 -> [w482 w488]
            tunnel: w465 -> [w483 w487]
            frame False {
              w480 = u16 2 items=["Default", "Pass Set Point", "Reset"] ("Menu Ring")
              n169 = call "injector setpoint.vi"("error in (no error)"=w483, "Pass setpoint?"=w480, "VISA Refnum in"=w482) -> ("error out"=w484:errorcluster, "MFC options"=w486:u16, "VISA Refnum out"=w485:refnum<visa-resource-name>)  [unwired: 6 in]
              n170 = property on="Set point (slpm)" class="DigNum (strict)"("Value"=0.0 ("Set point (slpm)")) -> ()  [unwired: 2 in, 2 out]
              n171 = property on="Inj. options" class="Ring (strict)"("Value"=w486) -> ()  [unwired: 2 in, 2 out]
            }
            frame True {
              n172 = property on="Set point (slpm)" class="DigNum (strict)"() -> ("Value"=w493:dbl)  [unwired: 2 in, 2 out]
              n173 = property on="Inj. options" class="Ring (strict)"() -> ("Value"=w490:u16)  [unwired: 2 in, 2 out]
              n174 = call "injector setpoint.vi"("error in (no error)"=w487, "set point"=w493, "Pass setpoint?"=w490, "VISA Refnum in"=w488) -> ("error out"=w491:errorcluster, "MFC options"=w489:u16, "VISA Refnum out"=w492:refnum<visa-resource-name>)  [unwired: 5 in]
              n175 = property on="Inj. options" class="Ring (strict)"("Value"=w489) -> ()  [unwired: 2 in, 2 out]
            }
          }
          n176 = call "Alicat_command case v2.vi"("Case"=T7."Poll", "error in (no error)"=w475, "VISA resource name"=w476) -> ("error out"=w473:errorcluster, "String From Alicat"=w472:string, "dup VISA resource name"=w463:refnum<visa-resource-name>)  [unwired: 5 in, 1 out]
          n177 = call "parse by space_v2019_07_18.vi"("error in (no error)"=w473, "String"=w472) -> ("error out"=w464:errorcluster, "Array"=w471:string[])  [unwired: 8 in]
          n178 = call "injector string unpack.vi"("lower limit"="lower limit", "upper limit"="upper limit", "Array"=w471) -> ("write data?"=→"write inj data?":bool, "data out"=→"injector data":T5, "mass flow/setpoint"=w460:cluster{"[4]":dbl, "[5]":dbl}, "pressure/temp"=→"Injector status":cluster{"[1]":dbl, "[2]":dbl}, "Temp In Range?"=w452:bool)  [unwired: 2 in, 2 out]
          n179 = Unbundle(w460) -> ("[4]"=→"mass flow (slpm)":dbl, "[5]"=→"set point (slpm)":dbl)
          n180 = Greater?(x=w451, y=w452) -> (0:w453:bool)
          n181 = case shown="False" w453 {
            tunnel: w452 -> [w478 w479]
            frame False {
              n182 = local write "Temp In Range?"(w478) -> ()
            }
            frame True {
              n183 = property on="Temp In Range?" class="Bool (strict)"("Val(Sgnl)"=w479) -> ()  [unwired: 2 in, 2 out]
            }
          }
          n184 = property on="Boolean" class="Bool (strict)"() -> ("Value"=w462:bool)  [unwired: 2 in, 2 out]
        }
        n185 = property on="Warming up" class="Bool (strict)"("Value"=FALSE ("Warming up")) -> ()  [unwired: 2 in, 2 out]
        n186 = call "check for csv filename.vi"("Canceled?"=w383, "selected path"=w390) -> ("file name"=→"file name":string, "Result path"=w386:path, "stripped path"=→"path":path)  [unwired: 7 in]
        "Result path" <- w386
        n187 = property on="Zeroing" class="Bool (strict)"("Value"=FALSE ("Zeroing")) -> ()  [unwired: 2 in, 2 out]
        n188 = while {
          tunnel: [w410] -> w387
          tunnel: w386 -> [w410]
          stop <- w407 stop-if-true
          n189 = property on="write inj data?" class="Bool (strict)"() -> ("Value"=w408:bool)  [unwired: 2 in, 2 out]
          n190 = property on="write GA data?" class="Bool (strict)"() -> ("Value"=w409:bool)  [unwired: 2 in, 2 out]
          n191 = And(x=w408, y=w409) -> (x .and. y?=w407:bool)
        }
        n192 = while {
          shift-right: [w445] -> _
          shift-left: w387 -> [w449]
          stop <- w420 stop-if-true
          n193 = property on="Base GA data" class="Clust (strict)"() -> ("Value"=w416:T1)  [unwired: 2 in, 2 out]
          n194 = property on="GA data" class="Clust (strict)"() -> ("Value"=w444:T1)  [unwired: 2 in, 2 out]
          n195 = property on="injector data" class="Clust (strict)"() -> ("Value"=w438:T5)  [unwired: 2 in, 2 out]
          n196 = Get Date/Time In Seconds() -> (seconds since 1Jan1904=w419:timestamp)
          n197 = Unbundle(w416) -> ("Array[3]"=w415:string, "Array[4]"=w414:string, "Array[7]"=w413:string, "Array[8]"=w412:string, "Array[9]"=w411:string)  [unwired: 3 out]
          n198 = Get Date/Time String(seconds (now)=w419, want seconds? (F)=TRUE) -> (date string=w422:string)  [unwired: 1 in, 1 out]
          n199 = Unbundle(w444) -> ("Array[3]"=w443:string, "Array[4]"=w442:string, "Array[7]"=w441:string, "Array[8]"=w440:string, "Array[9]"=w439:string)  [unwired: 3 out]
          n200 = Unbundle(w438) -> ("[1]"=w437:dbl, "[2]"=w436:dbl, "[3]"=w435:dbl, "[4]"=w434:dbl, "[5]"=w433:dbl)  [unwired: 3 out]
          n201 = property on="Result path" class="Path"() -> ("Value"=w448:path)  [unwired: 2 in, 2 out]
          n202 = Format Date/Time String(time format string (%c)="%H:%M:%S%3u", seconds (now)=w419) -> (date/time string=w417:string)  [unwired: 1 in]
          n203 = Build Array(w437, w436, w435, w434, w433) -> (w432:dbl[])
          n204 = Equal?(x=w449, y=w448) -> (x = y?=w450:bool)
          n205 = Select(t=w449, s=w450, f=w448) -> (s? t:f=w445:path)
          n206 = Number To Fractional String(number=w432) -> (F-format string=w431:string[])  [unwired: 3 in]
          n207 = Array To Cluster(array=w431) -> (cluster=w430:T9)
          n208 = Strip Path(path=w445) -> (stripped path=w446:path, name=w447:string)
          n209 = Unbundle(w430) -> ("[0]"=w429:string, "[1]"=w428:string, "[2]"=w427:string, "[3]"=w426:string, "[4]"=w425:string)
          n210 = property on="file name" class="Str"("Value"=w447) -> ()  [unwired: 2 in, 2 out]
          n211 = property on="path" class="Path"("Value"=w446) -> ()  [unwired: 2 in, 2 out]
          n212 = Build Array(w422, w417, w443, w442, w441, w440, w439, w422, w417, w429, w428, w427, w426, w425, w415, w414, w413, w412, w411) -> (w424:string[])
          n213 = call "Write Data_Header_v2.vi"("File path"=w445, "Array"=w424) -> ()  [unwired: 10 in]
          n214 = property on="Boolean" class="Bool (strict)"() -> ("Value"=w420:bool)  [unwired: 2 in, 2 out]
          n215 = Wait Until Next ms Multiple(millisecond multiple=u32 400) -> ()  [unwired: 1 out]
        }
        n216 = Select(t=T4."Shutdown" ("Enum"), s=w401, f=T4."Run" ("Enum")) -> (s? t:f=w400:T4)
      }
      frame "Shutdown" {
      }
    }
    "Current value" <- w51
    n217 = property on="Boolean" class="Bool (strict)"() -> ("Value"=w50:bool)  [unwired: 2 in, 2 out]
  }
  n218 = while {
    stop <- w562 stop-if-true
    n219 = event shown="[2] \"Estimated Flow (scfm)\", \"Target CO2 Concentration (ppm)\", \"Ambient CO2 (ppm)\", \"Actual Injection Rate (slpm)\", \"Actual Measured CO2 Concentration (ppm)\", \"Actual Baseline CO2 Concentration (ppm)\": Value Change" {
      selector: _ -> [_ _ _]
      dyn-events: _ -> [_ _ _]
      timeout: 100 -> [_ _ _]
      event Timeout {
        n220 = event-data() -> ()  [unwired: 1 in, 3 out]
      }
      event "Estimated Usable Weight (lbs)", "Injection rate (slpm)": Value Change {
        n221 = event-data() -> ()  [unwired: 1 in, 6 out]
        n222 = formula code="time = (massCO2 / (injRate * 0.00406)) * 60;"("massCO2"="Injection rate (slpm)", "injRate"="Estimated Usable Weight (lbs)") -> ("time"=→"Estimated test time avialable (hh:mm:ss)":dbl)
      }
      event "Estimated Flow (scfm)", "Target CO2 Concentration (ppm)", "Ambient CO2 (ppm)", "Actual Injection Rate (slpm)", "Actual Measured CO2 Concentration (ppm)", "Actual Baseline CO2 Concentration (ppm)": Value Change {
        n223 = event-data() -> ()  [unwired: 1 in, 6 out]
        n224 = formula code="float measuredAccCO2;\nfloat baselineAccCO2;\nfloat injUncert;\nfloat measuredUncert;\nfloat baselineUncert;\nfloat slpTOscf;\nfloat injFullScale;\nslpTOscf = 0.034854;\ninjFullScale = 500;\nif(measuredCO2 > 2000){\nmeasuredAccCO2 = 0.01 * measuredCO2;\n}\nelse {\nmeasuredAccCO2 = 20;\n}\nif(baselineCO2 > 2000){\nbaselineAccCO2 = baselineCO2 * 0.01;\n}\nelse{\nbaselineAccCO2 = 20;\n}\n\ncalFlow = ((mDotCO2 * slpTOscf * (10.** 6 - baselineCO2))/(measuredCO2 - baselineCO2))-(mDotCO2 * slpTOscf);\ninjUncert = ((((slpTOscf * (10. ** 6 - baselineCO2))/(measuredCO2 - baselineCO2))-slpTOscf)*((mDotCO2*0.004) + (injFullScale*0.002)));\nmeasuredUncert = ((-(slpTOscf * (10. ** 6 - baselineCO2) * mDotCO2)/(measuredCO2 - baselineCO2)**2)  * measuredAccCO2);\nbaselineUncert = (((slpTOscf * 10. ** 6 * mDotCO2)/(measuredCO2 - baselineCO2)**2) * baselineAccCO2);\nunCert = sqrt(injUncert ** 2 + measuredUncert ** 2 + baselineUncert ** 2);\npctUncert = (unCert / calFlow) * 100.;\n\nestMdotCO2 = estFlow / ( ((10**6 - baselineCO2)/(targetCO2 - ambientCO2)-1) * slpTOscf);"("targetCO2"="Target CO2 Concentration (ppm)", "ambientCO2"="Ambient CO2 (ppm)", "estFlow"="Estimated Flow (scfm)", "mDotCO2"="Actual Injection Rate (slpm)", "measuredCO2"="Actual Measured CO2 Concentration (ppm)", "baselineCO2"="Actual Baseline CO2 Concentration (ppm)") -> ("pctUncert"=→"Uncertainty (%)":dbl, "unCert"=→"Uncertainty (+/- scfm)":dbl, "calFlow"=→"Calculated Flow (scfm)":dbl, "estMdotCO2"=→"Estimated Injection Rate (slpm)":dbl)
      }
    }
    n225 = Wait (ms)(milliseconds to wait=u32 50) -> ()  [unwired: 1 out]
    n226 = property on="Boolean" class="Bool (strict)"() -> ("Value"=w562:bool)  [unwired: 2 in, 2 out]
  }
  n227 = while {
    stop <- w577 stop-if-true
    n228 = Wait (ms)(milliseconds to wait=u32 500 ("millisecond multiple")) -> ()  [unwired: 1 out]
    n229 = property on="Abort!" class="Bool (strict)"() -> ("Value"=w577:bool)  [unwired: 2 in, 2 out]
    n230 = Get Date/Time In Seconds() -> (seconds since 1Jan1904=→"Current time":timestamp)
  }
  n231 = while {
    stop <- w579 stop-if-true
    n232 = event shown="[1] \"Start new filename\": Value Change" {
      selector: _ -> [_ _]
      dyn-events: _ -> [_ _]
      timeout: 100 -> [_ _]
      event Timeout {
        n233 = event-data() -> ()  [unwired: 1 in, 3 out]
      }
      event "Start new filename": Value Change {
        n234 = event-data() -> ()  [unwired: 1 in, 5 out]
        n235 = call "Test file name2"() -> ("selected path"=w586:path, "cancelled"=w585:bool)  [unwired: 12 in, 2 out]
        n236 = call "check for csv filename.vi"("selected path"=w586) -> ("Result path"=w582:path)  [unwired: 8 in, 2 out]
        n237 = property on="Result path" class="Path"() -> ("Value"=w584:path)  [unwired: 2 in, 2 out]
        n238 = Select(t=w584, s=w585, f=w582) -> (s? t:f=w583:path)
        n239 = property on="Result path" class="Path"("Value"=w583) -> ()  [unwired: 2 in, 2 out]
      }
    }
    n240 = property on="Abort!" class="Bool (strict)"() -> ("Value"=w579:bool)  [unwired: 2 in, 2 out]
    n241 = Wait (ms)(milliseconds to wait=u32 50) -> ()  [unwired: 1 out]
  }
  n242 = while {
    stop <- w600 stop-if-true
    n243 = local read "Temp In Range?"() -> (w588:bool)
    n244 = property on="GA data" class="Clust (strict)"() -> ("Value"=w598:T1)  [unwired: 2 in, 2 out]
    n245 = property on="injector data" class="Clust (strict)"() -> ("Value"=w599:T5)  [unwired: 2 in, 2 out]
    n246 = property on="Base GA data" class="Clust (strict)"() -> ("Value"=w596:T1)  [unwired: 2 in, 2 out]
    n247 = Wait Until Next ms Multiple(millisecond multiple=u32 500) -> ()  [unwired: 1 out]
    n248 = while {
      tunnel: [w617] -> w592
      i -> [w616]
      stop <- w615 stop-if-true
      n249 = property on="write inj data?" class="Bool (strict)"() -> ("Value"=w620:bool)  [unwired: 2 in, 2 out]
      n250 = property on="write GA data?" class="Bool (strict)"() -> ("Value"=w619:bool)  [unwired: 2 in, 2 out]
      n251 = Get Date/Time In Seconds() -> (seconds since 1Jan1904=w617:timestamp)
      n252 = And(x=w620, y=w619) -> (x .and. y?=w615:bool)
      n253 = Greater Than 0?(x=w616) -> (x > 0?=w618:bool)
      n254 = And(x=w615, y=w618) -> (x .and. y?=w614:bool)
      n255 = case shown="True" w614 {
        tunnel: w617 -> [_ w623]
        frame False {
        }
        frame True {
          n256 = Get Date/Time String(seconds (now)=w623, want seconds? (F)=TRUE) -> (date string=w624:string)  [unwired: 1 in, 1 out]
          n257 = Fract/Exp String To Number(string=w624) -> (number=w621:dbl)  [unwired: 3 in, 1 out]
          n258 = property on="Gas analyzer chart" class="WFChart (strict)"("XScale.Minimum"=w621) -> ()  [unwired: 2 in, 2 out]
          n259 = property on="Injector chart" class="WFChart (strict)"("XScale.Minimum"=w621) -> ()  [unwired: 2 in, 2 out]
        }
      }
    }
    n260 = Unbundle(w599) -> ("[4]"=w609:dbl, "[5]"=w607:dbl)  [unwired: 6 out]
    n261 = Unbundle(w598) -> ("Array[3]"=w605:string)  [unwired: 7 out]
    n262 = Unbundle(w596) -> ("Array[3]"=w595:string)  [unwired: 7 out]
    n263 = case shown="False" w588 {
      frame False {
        n264 = for {
          N: 2 -> [_]
          tunnel: i32[] [2, 0] -> [w612] mode=indexing
          n265 = property on="Injector chart" class="WFChart (strict)"("DisabledEnum"=w612) -> ()  [unwired: 2 in, 2 out]
          n266 = Wait (ms)(milliseconds to wait=u32 150) -> ()  [unwired: 1 out]
        }
      }
      frame True {
      }
    }
    n267 = Build Array(w609) -> (w608:dbl[])
    n268 = Build Array(w607) -> (w606:dbl[])
    n269 = Build Array(w605) -> (w604:string[])
    n270 = Fract/Exp String To Number(string=w604) -> (number=w603:dbl[])  [unwired: 3 in, 1 out]
    n271 = Build Array(w595) -> (w594:string[])
    n272 = Fract/Exp String To Number(string=w594) -> (number=w593:dbl[])  [unwired: 3 in, 1 out]
    n273 = Bundle By Name("Y"=w608, "t0"=w592) -> (w601:waveform(dbl))  [unwired: 1 in]
    n274 = Bundle By Name("Y"=w606, "t0"=w592) -> (w602:waveform(dbl))  [unwired: 1 in]
    n275 = Bundle By Name("Y"=w603, "t0"=w592) -> (w591:waveform(dbl))  [unwired: 1 in]
    n276 = Bundle By Name("Y"=w593, "t0"=w592) -> (w590:waveform(dbl))  [unwired: 1 in]
    n277 = property on="Boolean" class="Bool (strict)"() -> ("Value"=w600:bool)  [unwired: 2 in, 2 out]
    n278 = Build Array(w591, w590) -> (→"Gas analyzer chart":waveform(dbl)[])
    n279 = Build Array(w601, w602) -> (→"Injector chart":waveform(dbl)[])
  }
  n280 = while {
    stop <- w628 stop-if-true
    n281 = event shown="[1] \"Temp In Range?\": Value Change" {
      selector: _ -> [_ _]
      dyn-events: _ -> [_ _]
      timeout: 100 -> [_ _]
      tunnel: [TRUE "Temp In Range?"] -> w626
      event Timeout {
        n282 = event-data() -> ()  [unwired: 1 in, 3 out]
      }
      event "Temp In Range?": Value Change {
        n283 = event-data() -> ()  [unwired: 1 in, 6 out]
      }
    }
    n284 = property on="Abort!" class="Bool (strict)"() -> ("Value"=w628:bool)  [unwired: 2 in, 2 out]
    n285 = case shown="False" w626 {
      frame False {
        n286 = local read "lower limit"() -> (w634:dbl)
        n287 = local read "Injector status"() -> (w636:cluster{"[1]":dbl, "[2]":dbl})
        n288 = Unbundle(w636) -> ("[2]"=w633:dbl)  [unwired: 1 out]
        n289 = Greater?(x=w634, y=w633) -> (0:w632:bool)
        n290 = Select(t="LOW", s=w632, f="HIGH") -> (s? t:f=w629:string)
        n291 = call "Build Text3"("limit"=w629, "temperature"=w633) -> ("Result"=w638:string, "error out"=w635:errorcluster)  [unwired: 12 in]
        n292 = call "Display Message to User3"("error in (no error)"=w635, "Enable"=TRUE, "Message"=w638) -> ()  [unwired: 7 in, 2 out]
      }
      frame True {
      }
    }
    n293 = Wait (ms)(milliseconds to wait=u32 50) -> ()  [unwired: 1 out]
  }
  n294 = VISA Close(VISA resource name=w26, error in (no error)=w25) -> ()  [unwired: 1 out]
  n295 = VISA Close(VISA resource name=w13, error in (no error)=w12) -> ()  [unwired: 1 out]
  n296 = VISA Close(VISA resource name=w24, error in (no error)=w23) -> ()  [unwired: 1 out]
  n297 = Initialize Array(0.0 ("element"), 1 ("dimension size")) -> (w1:dbl[])
  n298 = Initialize Array(0.0 ("element"), 1 ("dimension size")) -> (w3:dbl[])
  n299 = Initialize Array(0.0 ("element"), 1 ("dimension size")) -> (w2:dbl[])
  n300 = while {
    shift-right: [w647] -> _
    shift-left: w1 -> [w656]
    shift-right: [w648] -> _
    shift-left: w2 -> [w655]
    shift-right: [w649] -> _
    shift-left: w3 -> [w654]
    stop <- w653 stop-if-true
    n301 = case shown="False" "Get CO2 AVG" {
      tunnel: w656 -> [w659 w684]
      tunnel: w655 -> [w658 w683]
      tunnel: [w660 w676] -> w651
      tunnel: [w663 w675] -> w650
      tunnel: [w661 w674] -> w648
      tunnel: [w664 w673] -> w647
      frame False {
        n302 = local read "Reset AVG"() -> (w662:bool)
        n303 = case shown="True" w662 {
          tunnel: [w668 w671] -> w664
          tunnel: [w665 w670] -> w663
          tunnel: [w667 w671] -> w661
          tunnel: [w666 w670] -> w660
          tunnel: w659 -> [w668 _]
          tunnel: w658 -> [w667 _]
          frame False {
            n304 = call-poly <vilib>:"Mean.vi"("X"=w667) -> ("mean"=w666:dbl)  [unwired: 1 out]
            n305 = call-poly <vilib>:"Mean.vi"("X"=w668) -> ("mean"=w665:dbl)  [unwired: 1 out]
          }
          frame True {
            w670 = 0.0 ("mean")
            w671 = dbl[] []
            n306 = local write "CO2 AVG Size"(0 ("CO2 AVG Size")) -> ()
          }
        }
      }
      frame True {
        n307 = local read "CO2 Baseline (PPM)"() -> (w677:dbl)
        n308 = local read "CO2 (PPM)"() -> (w679:dbl)
        n309 = Array Subset(array=w684, index=0) -> (w680:dbl[])  [unwired: 1 in]
        n310 = Array Subset(array=w683, index=0) -> (w678:dbl[])  [unwired: 1 in]
        n311 = Build Array (concatenate)(w680, w679) -> (w673:dbl[])
        n312 = Build Array (concatenate)(w678, w677) -> (w674:dbl[])
        n313 = Array Size(array=w673) -> (size(s)=→"CO2 AVG Size":i32)
        n314 = call-poly <vilib>:"Mean.vi"("X"=w673) -> ("mean"=w675:dbl)  [unwired: 1 out]
        n315 = call-poly <vilib>:"Mean.vi"("X"=w674) -> ("mean"=w676:dbl)  [unwired: 1 out]
      }
    }
    n316 = case shown="False" "Get Ing AVG" {
      tunnel: w654 -> [w688 w698]
      tunnel: [w687 w699] -> w652
      tunnel: [w685 w695] -> w649
      frame False {
        n317 = case shown="True" "Reset AVG" {
          tunnel: w688 -> [w689 _]
          tunnel: [w690 0.0 ("mean")] -> w687
          tunnel: [w689 dbl[] [0.0]] -> w685
          frame False {
            n318 = call-poly <vilib>:"Mean.vi"("X"=w689) -> ("mean"=w690:dbl)  [unwired: 1 out]
          }
          frame True {
            n319 = local write "Ing AVG Size"(0 ("Ing AVG Size")) -> ()
          }
        }
      }
      frame True {
        n320 = local read "mass flow (slpm)"() -> (w700:dbl)
        n321 = Array Subset(array=w698, index=0) -> (w697:dbl[])  [unwired: 1 in]
        n322 = Build Array (concatenate)(w697, w700) -> (w695:dbl[])
        n323 = Array Size(array=w695) -> (size(s)=→"Ing AVG Size":i32)
        n324 = call-poly <vilib>:"Mean.vi"("X"=w695) -> ("mean"=w699:dbl)  [unwired: 1 out]
      }
    }
    n325 = formula code="float slTOcf = 0.0348544;\nfloat airflow = 0;\n\nairflow = (mass_flow * slTOcf * (10 ** 6 - baseline)) / (injection - baseline) - (mass_flow * slTOcf);"("mass_flow"=w652, "baseline"=w651, "injection"=w650) -> ("airflow"=w646:dbl)
    "Airflow (SCFM)" <- w646
    n326 = Get Date/Time In Seconds() -> (seconds since 1Jan1904=w644:timestamp)
    n327 = Build Array(w646) -> (w645:dbl[])
    n328 = property on="Boolean" class="Bool (strict)"() -> ("Value"=w653:bool)  [unwired: 2 in, 2 out]
    n329 = Bundle By Name("Y"=w645, "t0"=w644) -> (→"Airflow":waveform(dbl))  [unwired: 1 in]
    n330 = Wait Until Next ms Multiple(millisecond multiple=u32 400) -> ()  [unwired: 1 out]
  }
  "Warming up" <- FALSE ("Warming up")
  "Zeroing" <- FALSE ("Zeroing")
  "Boolean" <- FALSE ("Boolean")
